vi "Hall Example.vi"() -> ()   [LabVIEW 2011]
uses:
  <vilib>/Platform/TimedLoop/XDataNode/timing_clust.ctl
  <vilib>/Platform/TimedLoop/XDataNode/nitl_modes.ctl
  <vilib>/Platform/TimedLoop/XDataNode/wakeup.ctl
  <vilib>/rvi/DataTransferAndStorage/Container/Common/niFpgaContainerState.ctl
  <vilib>/rvi/DataTransferAndStorage/Container/Common/niFpgaDataTypeControl.ctl
  <vilib>/rvi/DataTransferAndStorage/Container/Common/niFpgaContainerImplementationControl.ctl
  <vilib>/rvi/DataTransferAndStorage/Container/Common/niFpgaContainerArbitrationOptionsControl.ctl
  <vilib>/rvi/DataTransferAndStorage/Container/Common/niFpgaTransferTypeControl.ctl
  <vilib>/rvi/DataTransferAndStorage/Container/Common/niFpgaContainerInitializationParameters.ctl
  <vilib>/rvi/Memory/Memory_Types/niFpgaMemoryInterfaceConfiguration.ctl
  <vilib>/rvi/FIFO/Fifo_Types/niFpgaFifoControlLogicControl.ctl
  <vilib>/rvi/DataTransferAndStorage/Container/Common/niFpgaContainerMetaDataKey.ctl
  <userlib>/AES/FPGA/FPGA TypeDefs/aes_FullyCustomTeeth ActionEngine Enum.ctl
  <userlib>/_NI VeriStand FPGA Support/NI VeriStand RIO Library/Custom Device Components/Engine Simulation/Engine Simulation Globals.vi
  <userlib>/AES/FPGA/FPGA VIs/AES ECU Event Measurement - All Measurements.vi
  <vilib>/rvi/eio/common/nirviEmuTemplateMethod_errors.vi
  <vilib>/rvi/DataTransferAndStorage/Container/Common/niFpgaContainerGetUniqueNameForEmu.vi
  <vilib>/rvi/DataTransferAndStorage/Container/Common/niFpgaContainerSetEmuInfo.vi
  <vilib>/rvi/eio/common/nirviEmuReportErrorAndStop.vi
  <vilib>/rvi/FIFO/Fifo_Resource/nirvififoEmulationSetSize.vi
  <vilib>/Platform/TimedLoop/XDataNode/XDataNode.xnode
  <vilib>/eio/EIONode/EIONode.xnode
  <vilib>/rvi/LocalResourceManager/LocalResourceManager.xnode
  <vilib>/rvi/DataTransferAndStorage/Container/XNode/niFpgaContainer.xnode
  <vilib>/rvi/FIFO/Fifo_Resource/nirvififoEmulationWrite.vi
  <vilib>/rvi/FIFO/Fifo_Resource/nirvififoEmulationRead.vi
  <vilib>/Platform/TimedLoop/XDataNode/XDNodeRunTimeDep.lvlib
  <userlib>/AES/FPGA/AES FPGA.lvlib
panel:
  out "ECUEvent.IC 1.End Angle":u64
  out "ECUEvent.IC 2.End Angle":u64
  out "ECUEvent.IC 3.End Angle":u64
  out "ECUEvent.IC 4.End Angle":u64
  out "ECUEvent.IC 5.End Angle":u64
  out "ECUEvent.IC 6.End Angle":u64
  out "ECUEvent.IC 7.End Angle":u64
  out "ECUEvent.IC 8.End Angle":u64
  out "ECUEvent.IC 1.Time Duration":u32
  out "ECUEvent.IC 1.Start Angle":u64
  out "ECUEvent.IC 1.Angle Duration":u64
  out "ECUEvent.IC 2.Time Duration":u32
  out "ECUEvent.IC 2.Start Angle":u64
  out "ECUEvent.IC 2.Angle Duration":u64
  out "ECUEvent.IC 3.Time Duration":u32
  out "ECUEvent.IC 3.Start Angle":u64
  out "ECUEvent.IC 3.Angle Duration":u64
  out "ECUEvent.IC 4.Time Duration":u32
  out "ECUEvent.IC 4.Start Angle":u64
  out "ECUEvent.IC 4.Angle Duration":u64
  out "ECUEvent.IC 5.Time Duration":u32
  out "ECUEvent.IC 5.Start Angle":u64
  out "ECUEvent.IC 5.Angle Duration":u64
  out "ECUEvent.IC 6.Time Duration":u32
  out "ECUEvent.IC 6.Start Angle":u64
  out "ECUEvent.IC 6.Angle Duration":u64
  out "ECUEvent.IC 7.Time Duration":u32
  out "ECUEvent.IC 7.Start Angle":u64
  out "ECUEvent.IC 7.Angle Duration":u64
  out "ECUEvent.IC 8.Time Duration":u32
  out "ECUEvent.IC 8.Start Angle":u64
  out "ECUEvent.IC 8.Angle Duration":u64
  out "ECUEvent.FI 1.End Angle":u64
  out "ECUEvent.FI 2.End Angle":u64
  out "ECUEvent.FI 3.End Angle":u64
  out "ECUEvent.FI 4.End Angle":u64
  out "ECUEvent.FI 5.End Angle":u64
  out "ECUEvent.FI 6.End Angle":u64
  out "ECUEvent.FI 7.End Angle":u64
  out "ECUEvent.FI 8.End Angle":u64
  out "ECUEvent.FI 1.Time Duration":u32
  out "ECUEvent.FI 1.Start Angle":u64
  out "ECUEvent.FI 1.Angle Duration":u64
  out "ECUEvent.FI 2.Time Duration":u32
  out "ECUEvent.FI 2.Start Angle":u64
  out "ECUEvent.FI 2.Angle Duration":u64
  out "ECUEvent.FI 3.Time Duration":u32
  out "ECUEvent.FI 3.Start Angle":u64
  out "ECUEvent.FI 3.Angle Duration":u64
  out "ECUEvent.FI 4.Time Duration":u32
  out "ECUEvent.FI 4.Start Angle":u64
  out "ECUEvent.FI 4.Angle Duration":u64
  out "ECUEvent.FI 5.Time Duration":u32
  out "ECUEvent.FI 5.Start Angle":u64
  out "ECUEvent.FI 5.Angle Duration":u64
  out "ECUEvent.FI 6.Time Duration":u32
  out "ECUEvent.FI 6.Start Angle":u64
  out "ECUEvent.FI 6.Angle Duration":u64
  out "ECUEvent.FI 7.Time Duration":u32
  out "ECUEvent.FI 7.Start Angle":u64
  out "ECUEvent.FI 7.Angle Duration":u64
  out "ECUEvent.FI 8.Time Duration":u32
  out "ECUEvent.FI 8.Start Angle":u64
  out "ECUEvent.FI 8.Angle Duration":u64
  in  "FullyCustomTeeth.Cams.Cam1.First Rising?":bool
  in  "FullyCustomTeeth.Cams.Num Angles":u8=2
  in  "FullyCustomTeeth.Cams.Cam1.Offset":u64
  in  "FullyCustomTeeth.Cams.Cam2.Offset":u64
  in  "FullyCustomTeeth.Cams.Cam3.Offset":u64
  in  "FullyCustomTeeth.Cams.Cam4.Offset":u64
  in  "FullyCustomTeeth.Cams.Num Profiles":u8=1
  in  "FullyCustomTeeth.Cams.Cam2.First Rising?":bool
  in  "FullyCustomTeeth.Cams.Cam3.First Rising?":bool
  in  "FullyCustomTeeth.Cams.Cam4.First Rising?":bool
  in  "FullyCustomTeeth.Cams.Cam1.CycleAngle":bool=TRUE
  in  "FullyCustomTeeth.Cams.Cam2.CycleAngle":bool=TRUE
  in  "FullyCustomTeeth.Cams.Cam3.CycleAngle":bool=TRUE
  in  "FullyCustomTeeth.Cams.Cam4.CycleAngle":bool=TRUE
  in  "FullyCustomTeeth.Cams.Data":u64
  in  "FullyCustomTeeth.Cams.Toggle":bool
  in  "NTeeth.Crank.TDC Offset":u64
  in  "NTeeth.Crank.Degrees High Pulse":u64
  in  "NTeeth.Crank.Degrees Low Pulse":u64
  in  "NTeeth.Crank.Num Teeth Miss":u8=2 caption="Num. Crank Teeth Missing"
  in  "NTeeth.Crank.Missing Teeth Offset":u64
  in  "NTeeth.Crank.TopDeadCenter High?":bool=TRUE
  in  "NTeeth.Crank.CycleAngle":bool
  in  "APU.Degrees per Tick":u64
  out "APU.Crank Angle":u64
  out "APU.Cycle Angle":u64
  in  "APU.Reset":bool
  in  "APU.Increment Rate":u64
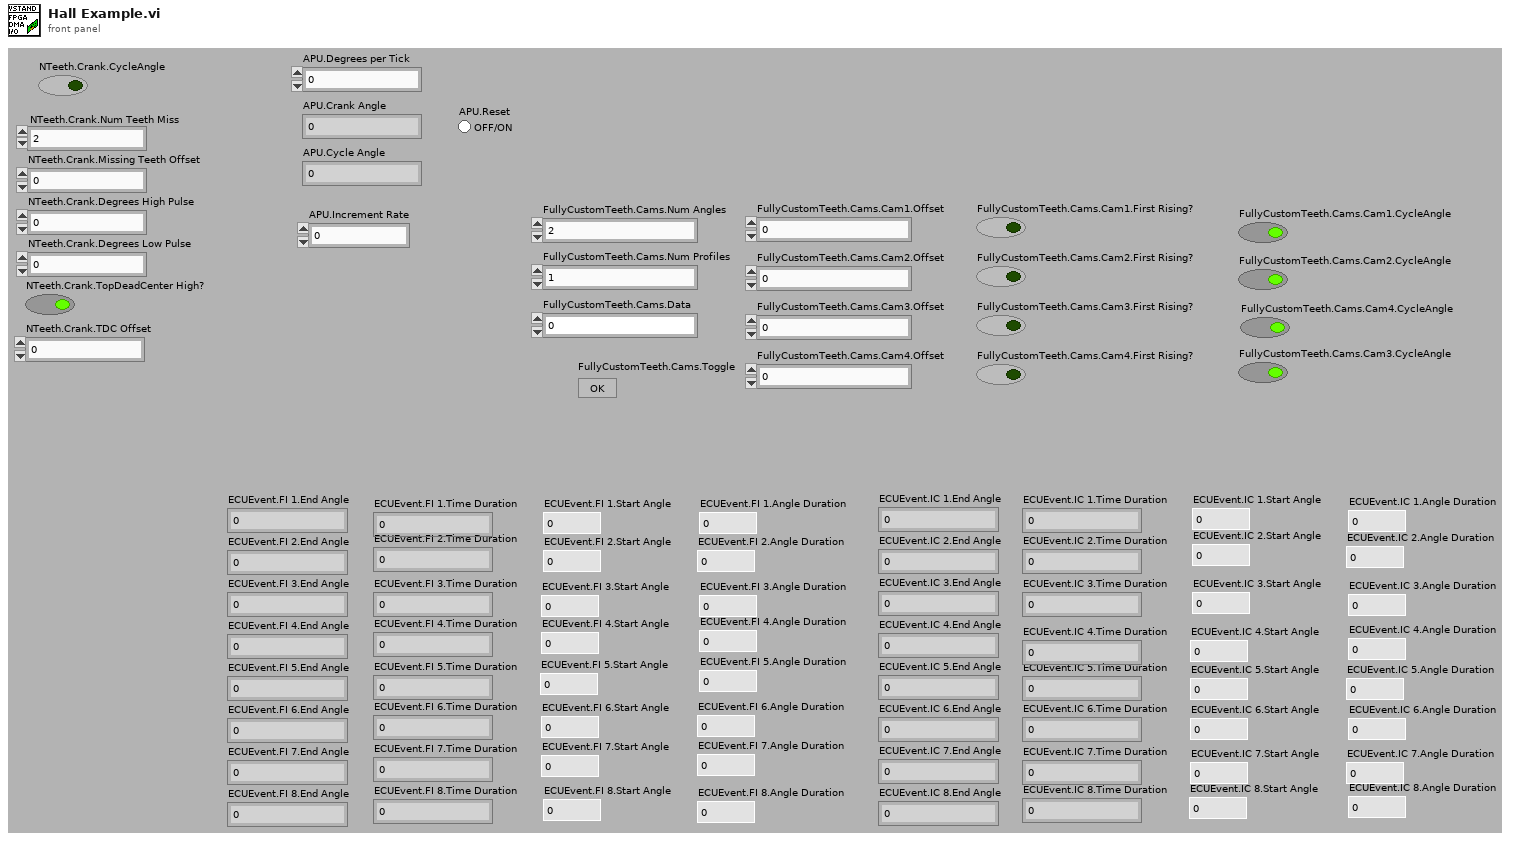
[diagram p1: front panel]
types:
  T1 = typedef "XDNodeRunTimeDep.lvlib/timing_clust.ctl" = cluster{"Expected End [f-1]":u64, "Actual End [f-1]":u64, "Finished Late? [f-1]":bool, "Expected End [i-1]":u64, "Actual End [i-1]":u64, "Finished Late? [i-1]":bool, "Expected Start [i]":u64, "Actual Start [i]":u64, "Expected Start [f]":u64, "Actual Start [f]":u64, "Source Name":string, "Structure Name":string, "Period":i64, "Deadline":i64, "Offset":i64, "Start":i64, "Priority":i32, "Timeout":i32, "Mode":T2, "Wakeup Reason":T3, "Error":errorcluster, "Source Type":string, "Secondary Source Type":string, "Global End Time":u64, "Global Start Time":u64, "Frame Duration":u64, "Iteration Duration":u64, "Assigned CPU":i32, "I/O Scan Engine Mode":u32}
  T2 = typedef "XDNodeRunTimeDep.lvlib/nitl_modes.ctl" = enum32{"No Change", "Process missed periods, maintain original phase", "Discard missed periods, maintain original phase", "Process missed periods, ignore original phase", "Discard missed periods, ignore original phase"}
  T3 = typedef "XDNodeRunTimeDep.lvlib/wakeup.ctl" = enum32{"Normal", "Aborted", "Asynchronous wakeup", "Timing source error", "Timed loop error", "Timeout"}
  T4 = typedef "AES.lvlib/AES FPGA.lvlib/aes_FullyCustomTeeth ActionEngine Enum.ctl" = enum16{"Write Angle", "Update Output"}
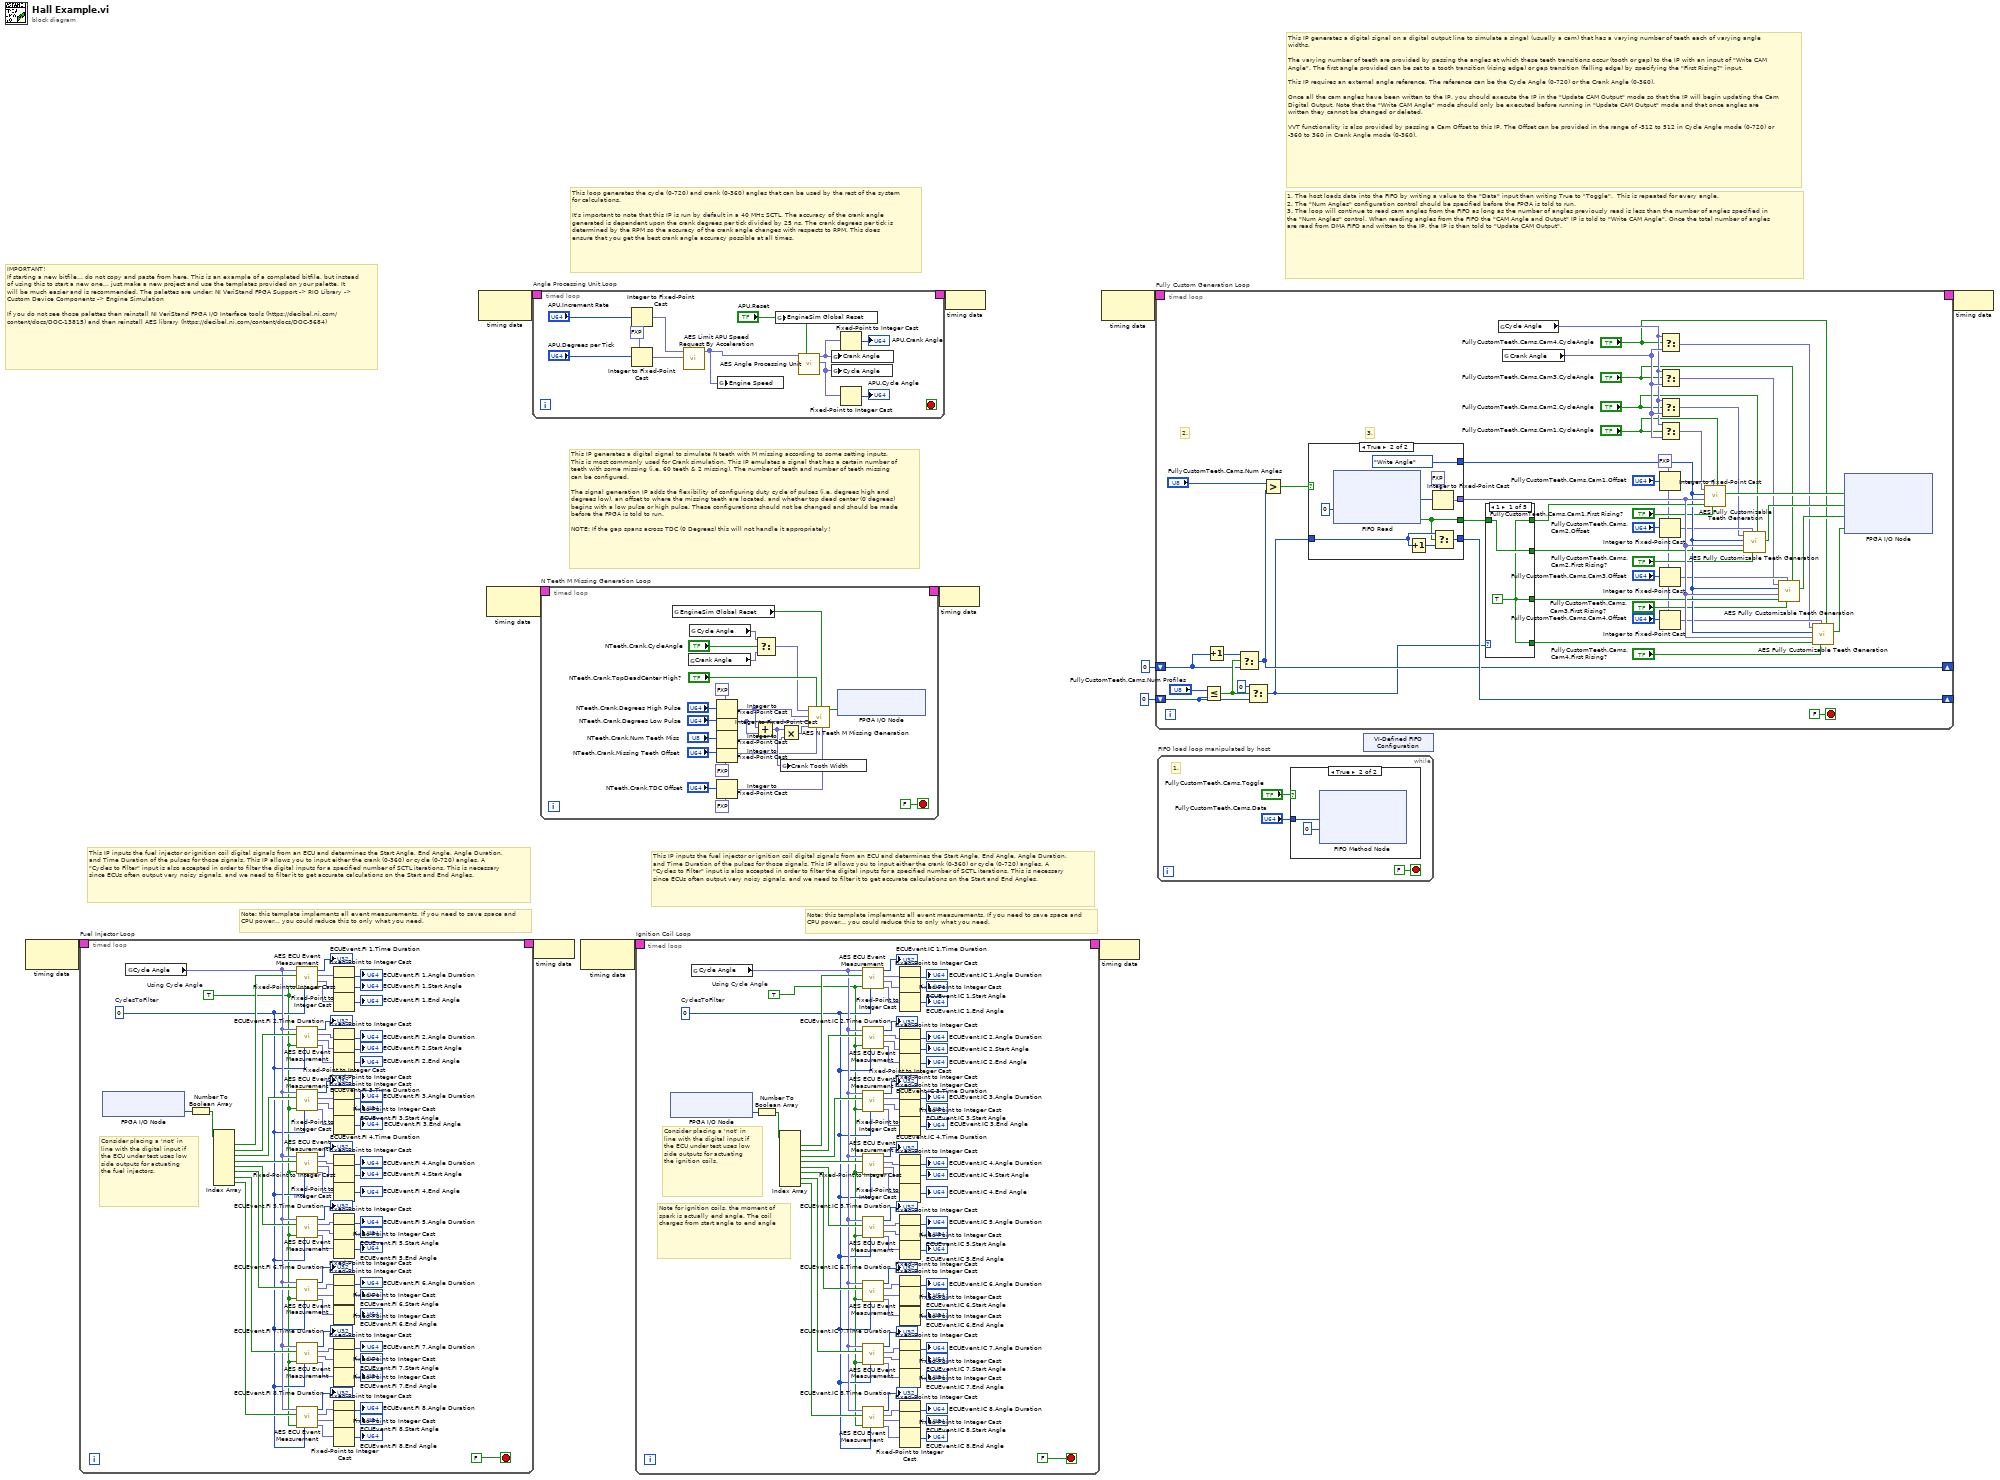
[diagram p0: block diagram]
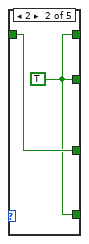
[diagram p3: hidden frame]
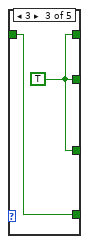
[diagram p4: hidden frame]
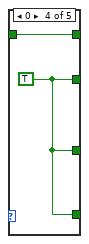
[diagram p5: hidden frame]
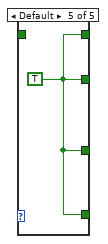
[diagram p6: hidden frame]
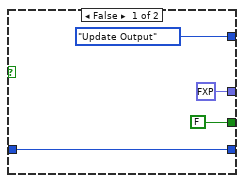
[diagram p7: hidden frame]
diagram:
  # "Note: this template implements all event measurements. If you need to save space and CPU power... you could reduce this to only what you need."
  # "This IP inputs the fuel injector or ignition coil digital signals from an ECU and determines the Start Angle, End Angle, Angle Duration, and Time Duration of the pulses for those signals. This IP allows you to input either the crank (0-360) or cycle (0-720) angles. A \"Cycles to Filter\" input is also accepted in order to filter the digital inputs for a specified number of SCTL iterations. This is necessary since ECUs often output very noisy signals, and we need to filter it to get accurate calculations on the Start and End Angles."
  # "Note: this template implements all event measurements. If you need to save space and CPU power... you could reduce this to only what you need."
  # "This IP inputs the fuel injector or ignition coil digital signals from an ECU and determines the Start Angle, End Angle, Angle Duration, and Time Duration of the pulses for those signals. This IP allows you to input either the crank (0-360) or cycle (0-720) angles. A \"Cycles to Filter\" input is also accepted in order to filter the digital inputs for a specified number of SCTL iterations. This is necessary since ECUs often output very noisy signals, and we need to filter it to get accurate calculations on the Start and End Angles."
  # "1. The host loads data into the FIFO by writing a value to the \"Data\" input then writing True to \"Toggle\".  This is repeated for every angle.\n2. The \"Num Angles\" configuration control should be specified before the FPGA is told to run.\n3. The loop will continue to read cam angles from the FIFO as long as the number of angles previously read is less than the number of angles specified in the \"Num Angles\" control. When reading angles from the FIFO the \"CAM Angle and Output\" IP is told to \"Write CAM Angle\". Once the total number of angles are read from DMA FIFO and written to the IP, the IP is then told to \"Update CAM Output\"."
  # "This IP generates a digital signal on a digital output line to simulate a singal (usually a cam) that has a varying number of teeth each of varying angle widths. \n\nThe varying number of teeth are provided by passing the angles at which these teeth transitions occur (tooth or gap) to the IP with an input of \"Write CAM Angle\". The first angle provided can be set to a tooth transition (rising edge) or gap transition (falling edge) by specifying the \"First Rising?\" input. \n\nThis IP requires an external angle reference. The reference can be the Cycle Angle (0-720) or the Crank Angle (0-360). \n\nOnce all the cam angles have been written to the IP, you should execute the IP in the \"Update CAM Output\" mode so that the IP will begin updating the Cam Digital Output. Note that the \"Write CAM Angle\" mode should only be executed before running in \"Update CAM Output\" mode and that once angles are written they cannot be changed or deleted.\n\nVVT functionality is also provided by passing a Cam Offset to this IP. The Offset can be provided in the range of -512 to 512 in Cycle Angle mode (0-720) or -360 to 360 in Crank Angle mode (0-360)."
  # "This IP generates a digital signal to simulate N teeth with M missing according to some setting inputs. This is most commonly used for Crank simulation. This IP emulates a signal that has a certain number of teeth with some missing (i.e. 60 teeth & 2 missing). The number of teeth and number of teeth missing can be configured. \n\nThe signal generation IP adds the flexibility of configuring duty cycle of pulses (i.e. degrees high and degrees low), an offset to where the missing teeth are located, and whether top dead center (0 degrees) begins with a low pulse or high pulse. These configurations should not be changed and should be made before the FPGA is told to run.\n\nNOTE: If the gap spans across TDC (0 Degrees) this will not handle it appropriately!"
  # "IMPORTANT!\nIf starting a new bitfile... do not copy and paste from here. This is an example of a completed bitfile, but instead of using this to start a new one... just make a new project and use the templates provided on your palette. It will be much easier and is recommended. The palettes are under: NI VeriStand FPGA Support -> RIO Library -> Custom Device Components -> Engine Simulation\n\nIf you do not see those palettes then reinstall NI VeriStand FPGA I/O Interface tools (https://decibel.ni.com/content/docs/DOC-13815) and then reinstall AES library (https://decibel.ni.com/content/docs/DOC-5684)"
  # "This loop generates the cycle (0-720) and crank (0-360) angles that can be used by the rest of the system for calculations. \n\nIt's important to note that this IP is run by default in a 40 MHz SCTL. The accuracy of the crank angle generated is dependent upon the crank degrees per tick divided by 25 ns. The crank degrees per tick is determined by the RPM so the accuracy of the crank angle changes with respects to RPM. This does ensure that you get the best crank angle accuracy possible at all times."
  n1 = node-c288() -> (w4:T1)  [unwired: 1 out]
  n2 = timed-loop "Fuel Injector Loop" {
    timing: w4 -> [_]
    timing-out: [_] -> w3
    stop <- FALSE stop-if-true
    w13 = TRUE  # Using Cycle Angle
    w71 = u16 0  # CyclesToFilter
    # "Consider placing a 'not' in line with the digital input if the ECU under test uses low side outputs for actuating the fuel injectors."
    n3 = xnode "FPGA I/O Node"() -> ("FuelInjector8:1"=w15:u8)  [unwired: 1 in, 1 out]
    n4 = global read "Engine Simulation Globals.vi" "Cycle Angle"() -> (w72:fxp<+,61,10>)
    n5 = Number To Boolean Array(number=w15) -> (Boolean array=w73:bool[])
    n6 = Index Array(array=w73) -> (element #1=w79:bool, element #2=w80:bool, element #3=w81:bool, element #4=w78:bool, element #5=w77:bool, element #6=w76:bool, element #7=w75:bool, element #8=w74:bool)  [unwired: 8 in]
    n7 = call-poly <userlib>:"AES ECU Event Measurement.vi"("Cycles to Filter"=w71, "Using Cycle Angle"=w13, "Digital Input Pulse"=w79, "Crank or Cyle Angle"=w72) -> ("End Angle (degrees)"=w62:fxp<+,61,10>, "Start Angle (degrees)"=w55:fxp<+,61,10>, "Angle Duration (degrees)"=w54:fxp<+/-,62,11>, "Time Duration (clock ticks)"=→"ECUEvent.FI 1.Time Duration":u32)  [unwired: 4 in]
    n8 = call-poly <userlib>:"AES ECU Event Measurement.vi"("Cycles to Filter"=w71, "Using Cycle Angle"=w13, "Digital Input Pulse"=w80, "Crank or Cyle Angle"=w72) -> ("End Angle (degrees)"=w61:fxp<+,61,10>, "Start Angle (degrees)"=w49:fxp<+,61,10>, "Angle Duration (degrees)"=w48:fxp<+/-,62,11>, "Time Duration (clock ticks)"=→"ECUEvent.FI 2.Time Duration":u32)  [unwired: 4 in]
    n9 = call-poly <userlib>:"AES ECU Event Measurement.vi"("Cycles to Filter"=w71, "Using Cycle Angle"=w13, "Digital Input Pulse"=w81, "Crank or Cyle Angle"=w72) -> ("End Angle (degrees)"=w60:fxp<+,61,10>, "Start Angle (degrees)"=w43:fxp<+,61,10>, "Angle Duration (degrees)"=w42:fxp<+/-,62,11>, "Time Duration (clock ticks)"=→"ECUEvent.FI 3.Time Duration":u32)  [unwired: 4 in]
    n10 = call-poly <userlib>:"AES ECU Event Measurement.vi"("Cycles to Filter"=w71, "Using Cycle Angle"=w13, "Digital Input Pulse"=w78, "Crank or Cyle Angle"=w72) -> ("End Angle (degrees)"=w59:fxp<+,61,10>, "Start Angle (degrees)"=w36:fxp<+,61,10>, "Angle Duration (degrees)"=w37:fxp<+/-,62,11>, "Time Duration (clock ticks)"=→"ECUEvent.FI 4.Time Duration":u32)  [unwired: 4 in]
    n11 = call-poly <userlib>:"AES ECU Event Measurement.vi"("Cycles to Filter"=w71, "Using Cycle Angle"=w13, "Digital Input Pulse"=w77, "Crank or Cyle Angle"=w72) -> ("End Angle (degrees)"=w58:fxp<+,61,10>, "Start Angle (degrees)"=w33:fxp<+,61,10>, "Angle Duration (degrees)"=w32:fxp<+/-,62,11>, "Time Duration (clock ticks)"=→"ECUEvent.FI 5.Time Duration":u32)  [unwired: 4 in]
    n12 = call-poly <userlib>:"AES ECU Event Measurement.vi"("Cycles to Filter"=w71, "Using Cycle Angle"=w13, "Digital Input Pulse"=w76, "Crank or Cyle Angle"=w72) -> ("End Angle (degrees)"=w29:fxp<+,61,10>, "Start Angle (degrees)"=w27:fxp<+,61,10>, "Angle Duration (degrees)"=w28:fxp<+/-,62,11>, "Time Duration (clock ticks)"=→"ECUEvent.FI 6.Time Duration":u32)  [unwired: 4 in]
    n13 = call-poly <userlib>:"AES ECU Event Measurement.vi"("Cycles to Filter"=w71, "Using Cycle Angle"=w13, "Digital Input Pulse"=w75, "Crank or Cyle Angle"=w72) -> ("End Angle (degrees)"=w57:fxp<+,61,10>, "Start Angle (degrees)"=w22:fxp<+,61,10>, "Angle Duration (degrees)"=w23:fxp<+/-,62,11>, "Time Duration (clock ticks)"=→"ECUEvent.FI 7.Time Duration":u32)  [unwired: 4 in]
    n14 = call-poly <userlib>:"AES ECU Event Measurement.vi"("Cycles to Filter"=w71, "Using Cycle Angle"=w13, "Digital Input Pulse"=w74, "Crank or Cyle Angle"=w72) -> ("End Angle (degrees)"=w56:fxp<+,61,10>, "Start Angle (degrees)"=w18:fxp<+,61,10>, "Angle Duration (degrees)"=w17:fxp<+/-,62,11>, "Time Duration (clock ticks)"=→"ECUEvent.FI 8.Time Duration":u32)  [unwired: 4 in]
    n15 = Fixed-Point to Integer Cast(1:w54) -> (0:→"ECUEvent.FI 1.Angle Duration":i64)
    n16 = Fixed-Point to Integer Cast(1:w55) -> (0:→"ECUEvent.FI 1.Start Angle":u64)
    n17 = Fixed-Point to Integer Cast(1:w62) -> (0:→"ECUEvent.FI 1.End Angle":u64)
    n18 = Fixed-Point to Integer Cast(1:w48) -> (0:→"ECUEvent.FI 2.Angle Duration":i64)
    n19 = Fixed-Point to Integer Cast(1:w49) -> (0:→"ECUEvent.FI 2.Start Angle":u64)
    n20 = Fixed-Point to Integer Cast(1:w61) -> (0:→"ECUEvent.FI 2.End Angle":u64)
    n21 = Fixed-Point to Integer Cast(1:w42) -> (0:→"ECUEvent.FI 3.Angle Duration":i64)
    n22 = Fixed-Point to Integer Cast(1:w43) -> (0:→"ECUEvent.FI 3.Start Angle":u64)
    n23 = Fixed-Point to Integer Cast(1:w60) -> (0:→"ECUEvent.FI 3.End Angle":u64)
    n24 = Fixed-Point to Integer Cast(1:w37) -> (0:→"ECUEvent.FI 4.Angle Duration":i64)
    n25 = Fixed-Point to Integer Cast(1:w36) -> (0:→"ECUEvent.FI 4.Start Angle":u64)
    n26 = Fixed-Point to Integer Cast(1:w59) -> (0:→"ECUEvent.FI 4.End Angle":u64)
    n27 = Fixed-Point to Integer Cast(1:w32) -> (0:→"ECUEvent.FI 5.Angle Duration":i64)
    n28 = Fixed-Point to Integer Cast(1:w33) -> (0:→"ECUEvent.FI 5.Start Angle":u64)
    n29 = Fixed-Point to Integer Cast(1:w58) -> (0:→"ECUEvent.FI 5.End Angle":u64)
    n30 = Fixed-Point to Integer Cast(1:w28) -> (0:→"ECUEvent.FI 6.Angle Duration":i64)
    n31 = Fixed-Point to Integer Cast(1:w27) -> (0:→"ECUEvent.FI 6.Start Angle":u64)
    n32 = Fixed-Point to Integer Cast(1:w29) -> (0:→"ECUEvent.FI 6.End Angle":u64)
    n33 = Fixed-Point to Integer Cast(1:w23) -> (0:→"ECUEvent.FI 7.Angle Duration":i64)
    n34 = Fixed-Point to Integer Cast(1:w22) -> (0:→"ECUEvent.FI 7.Start Angle":u64)
    n35 = Fixed-Point to Integer Cast(1:w57) -> (0:→"ECUEvent.FI 7.End Angle":u64)
    n36 = Fixed-Point to Integer Cast(1:w17) -> (0:→"ECUEvent.FI 8.Angle Duration":i64)
    n37 = Fixed-Point to Integer Cast(1:w18) -> (0:→"ECUEvent.FI 8.Start Angle":u64)
    n38 = Fixed-Point to Integer Cast(1:w56) -> (0:→"ECUEvent.FI 8.End Angle":u64)
  }
  n39 = node-c288() -> (w12:T1)  [unwired: 1 in]
  n40 = node-c288() -> (w10:T1)  [unwired: 1 out]
  n41 = timed-loop "Angle Processing Unit Loop" {
    timing: w12 -> [_]
    timing-out: [_] -> w11
    stop <- _ stop-if-true
    w87 = fxp<+/-,47,-4> 0.0 ("Crank.Degrees per Tick")
    n42 = Integer to Fixed-Point Cast(fixed-point type=w87, integer="APU.Increment Rate") -> (fixed-point=w86:fxp<+/-,47,-4>)
    n43 = Integer to Fixed-Point Cast(fixed-point type=w87, integer="APU.Degrees per Tick") -> (fixed-point=w89:fxp<+/-,47,-4>)
    n44 = call <userlib>:"AES Limit APU Speed Request By Acceleration.vi"("APU.Degrees per Tick in"=w89, "APU.Increment Rate"=w86) -> ("APU.Degrees per Tick out"=w85:fxp<+/-,47,-4>)  [unwired: 9 in]
    n45 = global write "Engine Simulation Globals.vi" "Engine Speed"(w85) -> ()
    n46 = global write "Engine Simulation Globals.vi" "EngineSim Global Reset"("APU.Reset") -> ()
    n47 = call <userlib>:"AES Angle Processing Unit.vi"("APU.Reset"="APU.Reset", "APU.Degrees per Tick"=w85) -> ("APU.Cycle Angle"=w91:fxp<+,61,10>, "APU.Crank Angle"=w95:fxp<+,60,9>)  [unwired: 8 in]
    n48 = global write "Engine Simulation Globals.vi" "Crank Angle"(w95) -> ()
    n49 = global write "Engine Simulation Globals.vi" "Cycle Angle"(w91) -> ()
    n50 = Fixed-Point to Integer Cast(1:w95) -> (0:→"APU.Crank Angle":u64)
    n51 = Fixed-Point to Integer Cast(1:w91) -> (0:→"APU.Cycle Angle":u64)
  }
  n52 = node-c288(w3) -> ()
  n53 = timed-loop "N Teeth M Missing Generation Loop" {
    timing: w10 -> [_]
    timing-out: [_] -> w9
    stop <- FALSE stop-if-true
    w115 = fxp<+,60,9> 0.0 ("NTeeth.Crank.Degrees High Pulse")
    n54 = global read "Engine Simulation Globals.vi" "EngineSim Global Reset"() -> (w102:bool)
    n55 = global read "Engine Simulation Globals.vi" "Crank Angle"() -> (w100:fxp<+,60,9>)
    n56 = global read "Engine Simulation Globals.vi" "Cycle Angle"() -> (w99:fxp<+,61,10>)
    n57 = Integer to Fixed-Point Cast(fixed-point type=w115, integer="NTeeth.Crank.Degrees High Pulse") -> (fixed-point=w107:fxp<+,60,9>)
    n58 = Integer to Fixed-Point Cast(fixed-point type=w115, integer="NTeeth.Crank.Degrees Low Pulse") -> (fixed-point=w109:fxp<+,60,9>)
    n59 = Integer to Fixed-Point Cast(integer="NTeeth.Crank.Num Teeth Miss") -> (fixed-point=w114:fxp<+,8,8>)  [unwired: 1 in]
    n60 = Integer to Fixed-Point Cast(fixed-point type=fxp<+,61,10> 0.0 ("NTeeth.Crank.Missing Teeth Offset"), integer="NTeeth.Crank.Missing Teeth Offset") -> (fixed-point=w110:fxp<+,61,10>)
    n61 = Integer to Fixed-Point Cast(fixed-point type=fxp<+/-,61,10> 0.0 ("NTeeth.TDC Offset"), integer="NTeeth.Crank.TDC Offset") -> (fixed-point=w103:fxp<+/-,61,10>)
    n62 = Add(x=w107, y=w109) -> (x+y=w118:fxp<+,61,10>)
    n63 = Select(t=w99, s="NTeeth.Crank.CycleAngle", f=w100) -> (s? t:f=w98:fxp<+,61,10>)
    n64 = Multiply(x=w118, y=w114) -> (x*y=w108:fxp<+,61,10>)
    n65 = global write "Engine Simulation Globals.vi" "Crank Tooth Width"(w118) -> ()
    n66 = call <userlib>:"AES N Teeth M Missing Generation.vi"("NTeeth.TDC Offset"=w103, "NTeeth.Reset"=w102, "NTeeth.Missing Teeth Offset"=w110, "NTeeth.TopDeadCenter High?"="NTeeth.Crank.TopDeadCenter High?", "NTeeth.Missing Teeth Gap"=w108, "NTeeth.Degrees Low Pulse"=w109, "NTeeth.Degrees High Pulse"=w107, "Crank or Cyle Angle"=w98) -> ("NTeeth.Digital Output"=w119:bool)  [unwired: 3 in]
    n67 = xnode "FPGA I/O Node"("CrankDigitalOut"=w119) -> ()  [unwired: 1 in, 1 out]
  }
  n68 = node-c288() -> (w2:T1)  [unwired: 1 out]
  n69 = timed-loop "Ignition Coil Loop" {
    timing: w2 -> [_]
    timing-out: [_] -> w1
    stop <- FALSE stop-if-true
    w123 = TRUE  # Using Cycle Angle
    w180 = u16 0  # CyclesToFilter
    # "Note for ignition coils, the moment of spark is actually end angle. The coil charges from start angle to end angle"
    # "Consider placing a 'not' in line with the digital input if the ECU under test uses low side outputs for actuating the ignition coils."
    n70 = xnode "FPGA I/O Node"() -> ("IgnitionCoil8:1"=w182:u8)  [unwired: 1 in, 1 out]
    n71 = global read "Engine Simulation Globals.vi" "Cycle Angle"() -> (w181:fxp<+,61,10>)
    n72 = Number To Boolean Array(number=w182) -> (Boolean array=w183:bool[])
    n73 = Index Array(array=w183) -> (element #1=w189:bool, element #2=w190:bool, element #3=w191:bool, element #4=w188:bool, element #5=w187:bool, element #6=w186:bool, element #7=w185:bool, element #8=w184:bool)  [unwired: 8 in]
    n74 = call-poly <userlib>:"AES ECU Event Measurement.vi"("Cycles to Filter"=w180, "Using Cycle Angle"=w123, "Digital Input Pulse"=w189, "Crank or Cyle Angle"=w181) -> ("End Angle (degrees)"=w171:fxp<+,61,10>, "Start Angle (degrees)"=w164:fxp<+,61,10>, "Angle Duration (degrees)"=w163:fxp<+/-,62,11>, "Time Duration (clock ticks)"=→"ECUEvent.IC 1.Time Duration":u32)  [unwired: 4 in]
    n75 = call-poly <userlib>:"AES ECU Event Measurement.vi"("Cycles to Filter"=w180, "Using Cycle Angle"=w123, "Digital Input Pulse"=w190, "Crank or Cyle Angle"=w181) -> ("End Angle (degrees)"=w170:fxp<+,61,10>, "Start Angle (degrees)"=w158:fxp<+,61,10>, "Angle Duration (degrees)"=w157:fxp<+/-,62,11>, "Time Duration (clock ticks)"=→"ECUEvent.IC 2.Time Duration":u32)  [unwired: 4 in]
    n76 = call-poly <userlib>:"AES ECU Event Measurement.vi"("Cycles to Filter"=w180, "Using Cycle Angle"=w123, "Digital Input Pulse"=w191, "Crank or Cyle Angle"=w181) -> ("End Angle (degrees)"=w169:fxp<+,61,10>, "Start Angle (degrees)"=w152:fxp<+,61,10>, "Angle Duration (degrees)"=w151:fxp<+/-,62,11>, "Time Duration (clock ticks)"=→"ECUEvent.IC 3.Time Duration":u32)  [unwired: 4 in]
    n77 = call-poly <userlib>:"AES ECU Event Measurement.vi"("Cycles to Filter"=w180, "Using Cycle Angle"=w123, "Digital Input Pulse"=w188, "Crank or Cyle Angle"=w181) -> ("End Angle (degrees)"=w168:fxp<+,61,10>, "Start Angle (degrees)"=w145:fxp<+,61,10>, "Angle Duration (degrees)"=w146:fxp<+/-,62,11>, "Time Duration (clock ticks)"=→"ECUEvent.IC 4.Time Duration":u32)  [unwired: 4 in]
    n78 = call-poly <userlib>:"AES ECU Event Measurement.vi"("Cycles to Filter"=w180, "Using Cycle Angle"=w123, "Digital Input Pulse"=w187, "Crank or Cyle Angle"=w181) -> ("End Angle (degrees)"=w167:fxp<+,61,10>, "Start Angle (degrees)"=w142:fxp<+,61,10>, "Angle Duration (degrees)"=w141:fxp<+/-,62,11>, "Time Duration (clock ticks)"=→"ECUEvent.IC 5.Time Duration":u32)  [unwired: 4 in]
    n79 = call-poly <userlib>:"AES ECU Event Measurement.vi"("Cycles to Filter"=w180, "Using Cycle Angle"=w123, "Digital Input Pulse"=w186, "Crank or Cyle Angle"=w181) -> ("End Angle (degrees)"=w138:fxp<+,61,10>, "Start Angle (degrees)"=w136:fxp<+,61,10>, "Angle Duration (degrees)"=w137:fxp<+/-,62,11>, "Time Duration (clock ticks)"=→"ECUEvent.IC 6.Time Duration":u32)  [unwired: 4 in]
    n80 = call-poly <userlib>:"AES ECU Event Measurement.vi"("Cycles to Filter"=w180, "Using Cycle Angle"=w123, "Digital Input Pulse"=w185, "Crank or Cyle Angle"=w181) -> ("End Angle (degrees)"=w166:fxp<+,61,10>, "Start Angle (degrees)"=w131:fxp<+,61,10>, "Angle Duration (degrees)"=w132:fxp<+/-,62,11>, "Time Duration (clock ticks)"=→"ECUEvent.IC 7.Time Duration":u32)  [unwired: 4 in]
    n81 = call-poly <userlib>:"AES ECU Event Measurement.vi"("Cycles to Filter"=w180, "Using Cycle Angle"=w123, "Digital Input Pulse"=w184, "Crank or Cyle Angle"=w181) -> ("End Angle (degrees)"=w165:fxp<+,61,10>, "Start Angle (degrees)"=w127:fxp<+,61,10>, "Angle Duration (degrees)"=w126:fxp<+/-,62,11>, "Time Duration (clock ticks)"=→"ECUEvent.IC 8.Time Duration":u32)  [unwired: 4 in]
    n82 = Fixed-Point to Integer Cast(1:w163) -> (0:→"ECUEvent.IC 1.Angle Duration":i64)
    n83 = Fixed-Point to Integer Cast(1:w164) -> (0:→"ECUEvent.IC 1.Start Angle":u64)
    n84 = Fixed-Point to Integer Cast(1:w171) -> (0:→"ECUEvent.IC 1.End Angle":u64)
    n85 = Fixed-Point to Integer Cast(1:w157) -> (0:→"ECUEvent.IC 2.Angle Duration":i64)
    n86 = Fixed-Point to Integer Cast(1:w158) -> (0:→"ECUEvent.IC 2.Start Angle":u64)
    n87 = Fixed-Point to Integer Cast(1:w170) -> (0:→"ECUEvent.IC 2.End Angle":u64)
    n88 = Fixed-Point to Integer Cast(1:w151) -> (0:→"ECUEvent.IC 3.Angle Duration":i64)
    n89 = Fixed-Point to Integer Cast(1:w152) -> (0:→"ECUEvent.IC 3.Start Angle":u64)
    n90 = Fixed-Point to Integer Cast(1:w169) -> (0:→"ECUEvent.IC 3.End Angle":u64)
    n91 = Fixed-Point to Integer Cast(1:w146) -> (0:→"ECUEvent.IC 4.Angle Duration":i64)
    n92 = Fixed-Point to Integer Cast(1:w145) -> (0:→"ECUEvent.IC 4.Start Angle":u64)
    n93 = Fixed-Point to Integer Cast(1:w168) -> (0:→"ECUEvent.IC 4.End Angle":u64)
    n94 = Fixed-Point to Integer Cast(1:w141) -> (0:→"ECUEvent.IC 5.Angle Duration":i64)
    n95 = Fixed-Point to Integer Cast(1:w142) -> (0:→"ECUEvent.IC 5.Start Angle":u64)
    n96 = Fixed-Point to Integer Cast(1:w167) -> (0:→"ECUEvent.IC 5.End Angle":u64)
    n97 = Fixed-Point to Integer Cast(1:w137) -> (0:→"ECUEvent.IC 6.Angle Duration":i64)
    n98 = Fixed-Point to Integer Cast(1:w136) -> (0:→"ECUEvent.IC 6.Start Angle":u64)
    n99 = Fixed-Point to Integer Cast(1:w138) -> (0:→"ECUEvent.IC 6.End Angle":u64)
    n100 = Fixed-Point to Integer Cast(1:w132) -> (0:→"ECUEvent.IC 7.Angle Duration":i64)
    n101 = Fixed-Point to Integer Cast(1:w131) -> (0:→"ECUEvent.IC 7.Start Angle":u64)
    n102 = Fixed-Point to Integer Cast(1:w166) -> (0:→"ECUEvent.IC 7.End Angle":u64)
    n103 = Fixed-Point to Integer Cast(1:w126) -> (0:→"ECUEvent.IC 8.Angle Duration":i64)
    n104 = Fixed-Point to Integer Cast(1:w127) -> (0:→"ECUEvent.IC 8.Start Angle":u64)
    n105 = Fixed-Point to Integer Cast(1:w165) -> (0:→"ECUEvent.IC 8.End Angle":u64)
  }
  n106 = node-c288(w9) -> ()
  n107 = node-c288(w11) -> ()
  n108 = node-c288(w1) -> ()
  n109 = node-c288() -> (w8:T1)  [unwired: 1 out]
  n110 = timed-loop "Fully Custom Generation Loop" {
    timing: w8 -> [_]
    timing-out: [_] -> w7
    shift-right: [w238] -> _
    shift-left: u8 0 -> [w231]
    shift-right: [w230] -> _
    shift-left: u8 0 ("CAM.Num Angles") -> [w232]
    stop <- FALSE stop-if-true
    w205 = fxp<+/-,61,10> 0.0 ("FullyCustomTeeth.Cams.Cam1.Offset")
    # "3."
    # "2."
    n111 = Less Or Equal?(x="FullyCustomTeeth.Cams.Num Profiles", y=w231) -> (x <= y?=w235:bool)
    n112 = Increment(x=w232) -> (x+1=w234:u8)
    n113 = Select(t=w234, s=w235, f=w232) -> (s? t:f=w230:u8)
    n114 = Select(t=u8 0, s=w235, f=w231) -> (s? t:f=w228:u8)
    n115 = Greater?(x="FullyCustomTeeth.Cams.Num Angles", y=w230) -> (0:w239:bool)
    n116 = case shown="True" w239 {
      tunnel: w228 -> [w253 w260]
      tunnel: [w253 w259] -> w238
      tunnel: [FALSE ("Timed Out?") w258] -> w227
      tunnel: [aes_FullyCustomTeeth_ActionEngine_Enum."Update Output" ("FullyCustomTeeth.Action") aes_FullyCustomTeeth_ActionEngine_Enum."Write Angle" ("FullyCustomTeeth.Action")] -> w218
      tunnel: [fxp<+,61,10> 0.0 ("Element") w255] -> w229
      frame False {
      }
      frame True {
        n117 = xnode ("FIFO Read")("Timeout"=0) -> ("Element"=w257:u64, "Timed Out?"=w258:bool)  [unwired: 1 in, 1 out]
        n118 = Increment(x=w260) -> (x+1=w261:u8)
        n119 = Integer to Fixed-Point Cast(fixed-point type=fxp<+,61,10> 0.0 ("Element"), integer=w257) -> (fixed-point=w255:fxp<+,61,10>)
        n120 = Select(t=w260, s=w258, f=w261) -> (s? t:f=w259:u8)
      }
    }
    n121 = case shown="1" w228 {
      tunnel: w227 -> [w242 w244 w245 w248 _]
      tunnel: [w241 w243 w246 w248 w249] -> w226
      tunnel: [w241 w244 w246 w247 w249] -> w224
      tunnel: [w242 w243 w246 w247 w249] -> w225
      tunnel: [w241 w243 w245 w247 w249] -> w223
      frame 1 {
        w241 = TRUE ("Timed Out?")
      }
      frame 2 {
        w243 = TRUE ("Timed Out?")
      }
      frame 3 {
        w246 = TRUE ("Timed Out?")
      }
      frame 0 {
        w247 = TRUE ("Timed Out?")
      }
      frame Default {
        w249 = TRUE ("Timed Out?")
      }
    }
    n122 = global read "Engine Simulation Globals.vi" "Cycle Angle"() -> (w203:fxp<+,61,10>)
    n123 = global read "Engine Simulation Globals.vi" "Crank Angle"() -> (w204:fxp<+,60,9>)
    n124 = Integer to Fixed-Point Cast(fixed-point type=w205, integer="FullyCustomTeeth.Cams.Cam1.Offset") -> (fixed-point=w212:fxp<+/-,61,10>)
    n125 = Integer to Fixed-Point Cast(fixed-point type=w205, integer="FullyCustomTeeth.Cams.Cam2.Offset") -> (fixed-point=w211:fxp<+/-,61,10>)
    n126 = Integer to Fixed-Point Cast(fixed-point type=w205, integer="FullyCustomTeeth.Cams.Cam3.Offset") -> (fixed-point=w208:fxp<+/-,61,10>)
    n127 = Integer to Fixed-Point Cast(fixed-point type=w205, integer="FullyCustomTeeth.Cams.Cam4.Offset") -> (fixed-point=w206:fxp<+/-,61,10>)
    n128 = Select(t=w203, s="FullyCustomTeeth.Cams.Cam4.CycleAngle", f=w204) -> (s? t:f=w195:fxp<+,61,10>)
    n129 = Select(t=w203, s="FullyCustomTeeth.Cams.Cam3.CycleAngle", f=w204) -> (s? t:f=w198:fxp<+,61,10>)
    n130 = Select(t=w203, s="FullyCustomTeeth.Cams.Cam2.CycleAngle", f=w204) -> (s? t:f=w200:fxp<+,61,10>)
    n131 = Select(t=w203, s="FullyCustomTeeth.Cams.Cam1.CycleAngle", f=w204) -> (s? t:f=w201:fxp<+,61,10>)
    n132 = call <userlib>:"AES Fully Customizable Teeth Generation.vi"("Using Cycle Angle"="FullyCustomTeeth.Cams.Cam1.CycleAngle", "FullyCustomTeeth.FirstElement RisingEdge?"="FullyCustomTeeth.Cams.Cam1.First Rising?", "FullyCustomTeeth.Offset"=w212, "Write Timeout?"=w226, "FullyCustomTeeth.Next Angle"=w229, "FullyCustomTeeth.Action"=w218, "Crank or Cyle Angle"=w201) -> ("FullyCustomTeeth.Digital Output"=w219:bool)  [unwired: 4 in]
    n133 = call <userlib>:"AES Fully Customizable Teeth Generation.vi"("Using Cycle Angle"="FullyCustomTeeth.Cams.Cam2.CycleAngle", "FullyCustomTeeth.FirstElement RisingEdge?"="FullyCustomTeeth.Cams.Cam2.First Rising?", "FullyCustomTeeth.Offset"=w211, "Write Timeout?"=w225, "FullyCustomTeeth.Next Angle"=w229, "FullyCustomTeeth.Action"=w218, "Crank or Cyle Angle"=w200) -> ("FullyCustomTeeth.Digital Output"=w220:bool)  [unwired: 4 in]
    n134 = call <userlib>:"AES Fully Customizable Teeth Generation.vi"("Using Cycle Angle"="FullyCustomTeeth.Cams.Cam3.CycleAngle", "FullyCustomTeeth.FirstElement RisingEdge?"="FullyCustomTeeth.Cams.Cam3.First Rising?", "FullyCustomTeeth.Offset"=w208, "Write Timeout?"=w224, "FullyCustomTeeth.Next Angle"=w229, "FullyCustomTeeth.Action"=w218, "Crank or Cyle Angle"=w198) -> ("FullyCustomTeeth.Digital Output"=w221:bool)  [unwired: 4 in]
    n135 = call <userlib>:"AES Fully Customizable Teeth Generation.vi"("Using Cycle Angle"="FullyCustomTeeth.Cams.Cam4.CycleAngle", "FullyCustomTeeth.FirstElement RisingEdge?"="FullyCustomTeeth.Cams.Cam4.First Rising?", "FullyCustomTeeth.Offset"=w206, "Write Timeout?"=w223, "FullyCustomTeeth.Next Angle"=w229, "FullyCustomTeeth.Action"=w218, "Crank or Cyle Angle"=w195) -> ("FullyCustomTeeth.Digital Output"=w222:bool)  [unwired: 4 in]
    n136 = xnode "FPGA I/O Node"("Cam1DigitalOut"=w219, "Cam2DigitalOut"=w220, "Cam3DigitalOut"=w221, "Cam4DigitalOut"=w222) -> ()  [unwired: 4 in, 4 out]
  }
  n137 = while "FIFO load loop manipulated by host" {
    stop <- FALSE stop-if-true
    # "1."
    n138 = case shown="True" "FullyCustomTeeth.Cams.Toggle" {
      tunnel: "FullyCustomTeeth.Cams.Data" -> [_ w269]
      frame False {
      }
      frame True {
        n139 = xnode ("FIFO Method Node")("Element"=w269, "Timeout"=0) -> ()  [unwired: 1 in, 2 out]
      }
    }
  }
  n140 = xnode "VI-Defined FIFO Configuration"() -> ()  [unwired: 1 out]
  n141 = node-c288(w7) -> ()
